vi "initRefUI.vi"(6 "main GUI Reference":refnum<vi>, 7 "Application Name":string, 8 "error in (no error)":errorcluster, 11 "guiTemplates in":refnum<class "stillnessHelper.lvclass">) -> (0 "error out":errorcluster, 3 "guiTemplates out":refnum<class "stillnessHelper.lvclass">, 4 "App Folder":path)   [LabVIEW 2022 SP3, in "stillnessHelper.lvclass"]
uses:
  stillnessHelper.lvclass
  stillnessHelper.lvclass/stillnessHelper.ctl
  <vilib>/Utility/sysdir.llb/System Directory Type.ctl
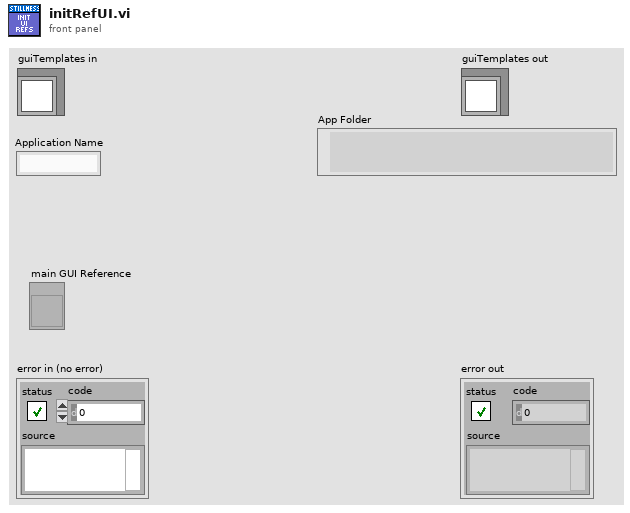
[diagram p1: front panel]
types:
  T1 = enum32{"invalid app kind", "Development System", "Run Time System", "Student Edition", "Embedded LabVIEW", "Evaluation", "Custom"}
  T2 = enum16{"Always On", "Always Off", "Off While Running"}
  T3 = typedef "System Directory Type.ctl" = i32
  T4 = enum32{"Invalid", "Standard", "Closed", "Hidden", "Minimized", "Maximized"}
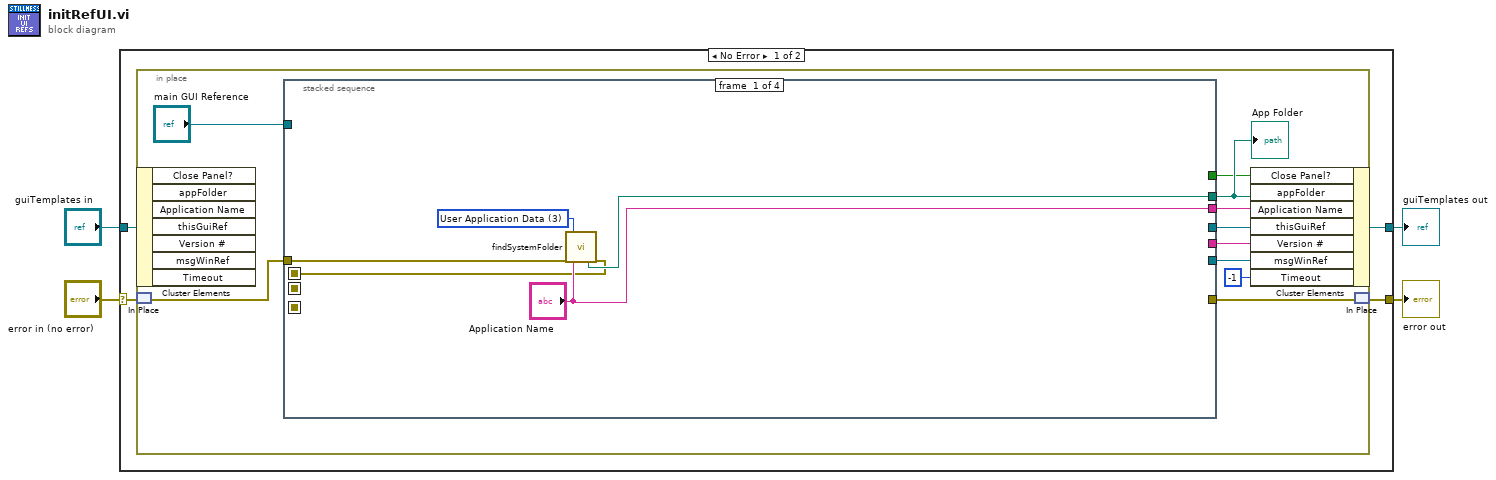
[diagram p0: block diagram]
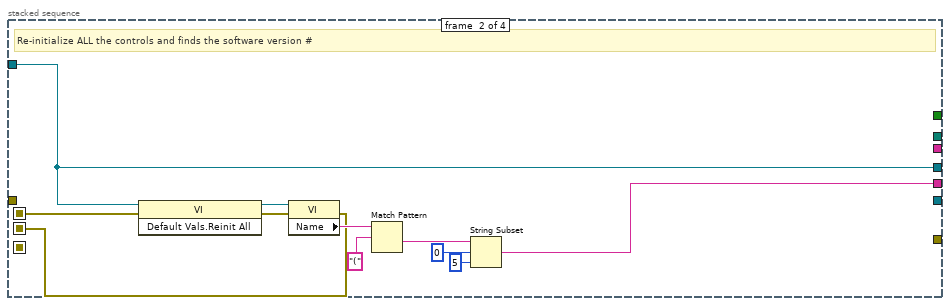
[diagram p2: hidden frame]
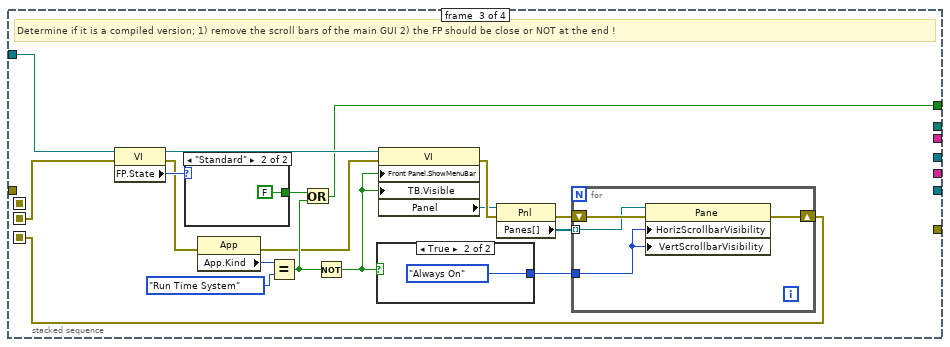
[diagram p3: hidden frame]
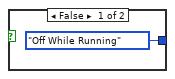
[diagram p4: hidden frame]
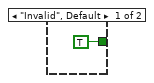
[diagram p5: hidden frame]
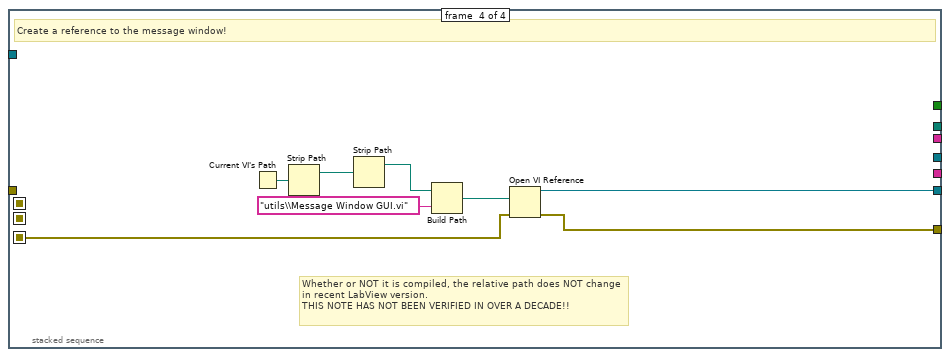
[diagram p6: hidden frame]
diagram:
  n1 = case shown="No Error" "error in (no error)" {
    selector: "error in (no error)" -> [w6 w70]
    tunnel: [w5 w70] -> w3
    tunnel: [w7 w69] -> w1
    tunnel: "guiTemplates in" -> [w8 w69]
    frame No Error {
      n2 = in-place {
        n3 = in-place-cluster #1(w8) -> ()  [unwired: 7 out]
        n4 = in-place-match #2(w6) -> (w18:errorcluster)
        n5 = stacked-sequence {
          seq-local: [w19 _ _ _] -> [_ w27 _ _]
          seq-local: [_ w26 _ _] -> [_ _ w37 _]
          seq-local: [_ _ w36 _] -> [_ _ _ w65]
          tunnel: w18 -> [w23 _ _ _]
          tunnel: ["Application Name" _ _ _] -> w17
          tunnel: [w20 _ _ _] -> w16
          tunnel: [_ w24 _ _] -> w15
          tunnel: [_ w25 _ _] -> w14
          tunnel: "main GUI Reference" -> [_ w25 w38 _]
          tunnel: [_ _ w35 _] -> w12
          tunnel: [_ _ _ w61] -> w11
          tunnel: [_ _ _ w64] -> w9
          frame #0 {
            w22 = T3 3 items=["User Home"=0, "User Desktop"=1, "User Documents"=2, "User Application Data"=3, "User Preferences"=4, "User Temporary"=5, "Public Documents"=6, "Public Application Data"=7, "Public Preferences"=8, "Public Cache"=13, "System Core Libraries"=9, "System Installed Libraries"=10, "Application Files"=11, "Boot Volume Root"=12] ("system directory type")
            n6 = call "findSystemFolder.vi"("error in (no error)"=w23, "system directory type"=w22, "Application Name"="Application Name") -> ("App Folder"=w20:path, "error out"=w19:errorcluster)  [unwired: 15 in]
          }
          frame #1 {
            # "Re-initialize ALL the controls and finds the software version #"
            n7 = invoke class="VI" method="Default Vals.Reinit All"(reference=w25, error in=w27) -> (reference out=w34:refnum<vi>, error out=w33:errorcluster)  [unwired: 1 in, 1 out]
            n8 = property class="VI"(reference=w34, error in=w33) -> (error out=w26:errorcluster, "Name"=w32:string)  [unwired: 1 out]
            n9 = Match Pattern(string=w32, regular expression="(") -> (after substring=w31:string)  [unwired: 1 in, 3 out]
            n10 = String Subset(string=w31, offset (0)=0, length (rest)=5 ("length (rest)")) -> (substring=w24:string)
          }
          frame #2 {
            # "Determine if it is a compiled version; 1) remove the scroll bars of the main GUI 2) the FP should be close or NOT at the end !"
            n11 = property class="VI"(reference=w38, error in=w37) -> (reference out=w44:refnum<vi>, error out=w41:errorcluster, "FP.State"=w42:T4)
            n12 = case shown="\"Standard\"" w42 {
              tunnel: [TRUE FALSE] -> w43
              frame "Invalid", Default {
              }
              frame "Standard" {
              }
            }
            n13 = property class="App"(error in=w41) -> (error out=w45:errorcluster, "App.Kind"=w40:T1)  [unwired: 1 in, 1 out]
            n14 = Equal?(x=w40, y=T1."Run Time System" ("Application:Kind")) -> (x = y?=w50:bool)
            n15 = Or(x=w43, y=w50) -> (x .or. y?=w35:bool)
            n16 = Not(x=w50) -> (.not. x?=w52:bool)
            n17 = case shown="True" w52 {
              tunnel: [T2."Off While Running" ("Horizontal Scrollbar Visibility") T2."Always On" ("Horizontal Scrollbar Visibility")] -> w51
              frame False {
              }
              frame True {
              }
            }
            n18 = property class="VI"(reference=w44, error in=w45, "Front Panel.ShowMenuBar"=w52, "TB.Visible"=w52) -> (error out=w47:errorcluster, "Panel"=w46:refnum<vi>)  [unwired: 1 out]
            n19 = property class="Pnl"(reference=w46, error in=w47) -> (error out=w48:errorcluster, "Panes[]"=w49:refnum<vi>[])  [unwired: 1 out]
            n20 = for {
              shift-right: [w57] -> w36
              shift-left: w48 -> [w58]
              tunnel: w49 -> [w56] mode=indexing
              tunnel: w51 -> [w55]
              n21 = property class="Pane"(reference=w56, error in=w58, "HorizScrollbarVisibility"=w55, "VertScrollbarVisibility"=w55) -> (error out=w57:errorcluster)  [unwired: 1 out]
            }
          }
          frame #3 {
            # "Whether or NOT it is compiled, the relative path does NOT change in recent LabView version.\nTHIS NOTE HAS NOT BEEN VERIFIED IN OVER A DECADE!!"
            # "Create a reference to the message window!"
            n22 = Current VI's Path() -> (path=w67:path)
            n23 = Strip Path(path=w67) -> (stripped path=w63:path)  [unwired: 1 out]
            n24 = Strip Path(path=w63) -> (stripped path=w62:path)  [unwired: 1 out]
            n25 = Build Path(base path=w62, name or relative path="utils\\Message Window GUI.vi") -> (appended path=w68:path)
            n26 = Open VI Reference(vi path=w68, error in (no error)=w65) -> (vi reference=w61:refnum<vi>, error out=w64:errorcluster)  [unwired: 4 in]
          }
        }
        "App Folder" <- w16
        n27 = in-place-cluster #1("Close Panel?"=w12, "appFolder"=w16, "Application Name"=w17, "thisGuiRef"=w14, "Version #"=w15, "msgWinRef"=w11, "Timeout"=-1 ("State Machine Control.Timeout")) -> (w7:refnum<class "stillnessHelper.lvclass">)
        n28 = in-place-match #2(w9) -> (w5:errorcluster)
      }
    }
    frame Error {
    }
  }
  "error out" <- w3
  "guiTemplates out" <- w1
